vi "Close.vi"(8 "error in (no error)":errorcluster, 11 "VISA resource name":refnum<visa-resource-name>) -> (0 "error out":errorcluster)   [LabVIEW 2012, in "Quantum Composers 9000 Series.lvlib"]
doc: "This VI unlocks the system keyboard and closes the I/O interface with the instrument."
uses:
  Quantum Composers 9000 Series.lvlib
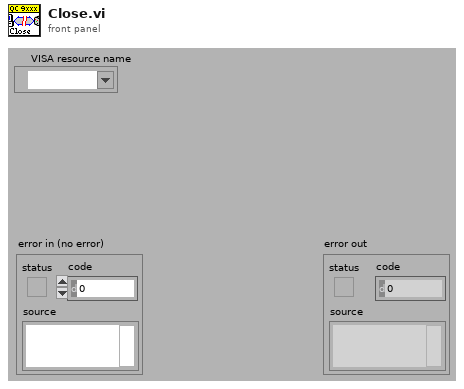
[diagram p1: front panel]
types:
  T1 = enum16{"Read Data", "Write Data", "Dispose of Data", "Clear ALL Data"}
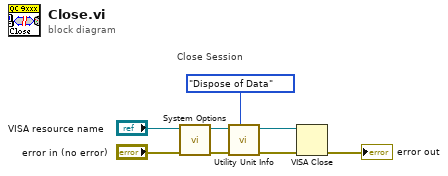
[diagram p0: block diagram]
diagram:
  # "Close Session"
  n1 = call "System Options.vi"("error in (no error)"="error in (no error)", "VISA resource name"="VISA resource name") -> ("error out"=w5:errorcluster, "VISA resource name out"=w4:refnum<visa-resource-name>)  [unwired: 5 in, 3 out]
  n2 = call "Utility Unit Info.vi"("Action"=T1."Dispose of Data", "Error In (no error)"=w5, "VISA resource name in"=w4) -> ("Error Out"=w2:errorcluster, "VISA resource name out"=w3:refnum<visa-resource-name>)  [unwired: 1 in, 6 out]
  n3 = VISA Close(VISA resource name=w3, error in (no error)=w2) -> (error out=→"error out":errorcluster)
